vi "KH_EthernetIPConfig_Globals.vi"() -> ()   [LabVIEW 2017]
uses:
  KH_EthernetIPConfig_TDef_Cluster_ConnectionParameter.ctl
panel:
  in  "EthernetIP_tab":enum32{"References"}(tab)
  in  "Ref Listbox ConfigItem":refnum<vi>
  in  "Ref Listbox Configuration":refnum<vi>
  in  "Table ConnectionManager":refnum<vi>
  in  "Ring ConnectionType":refnum<vi>
  in  "Ref Table Assembly":refnum<vi>
  in  "Cluster DeviceInformation":refnum<vi>
  in  "Ref Cluster ConnectionParam":refnum<vi>
  in  "Ref_ParamInputs":refnum<vi>
  # "Connection Type:"
  # "Priority:"
  # "Connection Type:"
  # "Priority:"
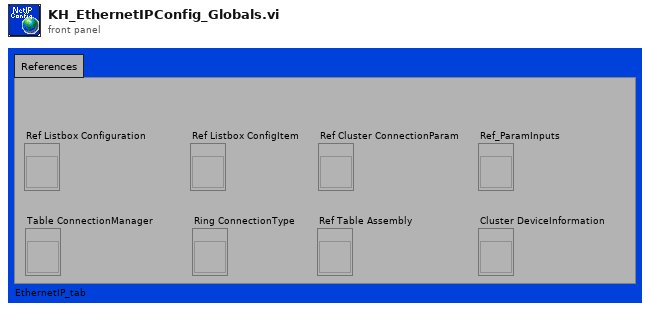
[diagram p1: front panel]
diagram:
